vi "Track Overflow.vi"(2 "reset":bool, 5 "overflow in":bool[](array[boolean])=[FALSE, FALSE, FALSE, FALSE, FALSE, FALSE, FALSE, FALSE, FALSE, FALSE, FALSE, FALSE, FALSE, FALSE, FALSE, FALSE], 7 "input valid":bool, 9 "latch overflow status":bool) -> (10 "overflow detected":bool)   [LabVIEW 2018, in "GettingStarted_5774_FPGA.lvlib"]
doc: "Tracks the overflow status.\n\nA rising edge on the <B>latch overflow status</B> input updates the <B>overflow detected</B> output: this output is set to true if an overflow was detected since the last update."
uses:
  GettingStarted_5774_FPGA.lvlib
  <instrlib>/_niInstr/Basic Elements/v1/FPGA/niInstr Basic Elements v1 FPGA.lvlib
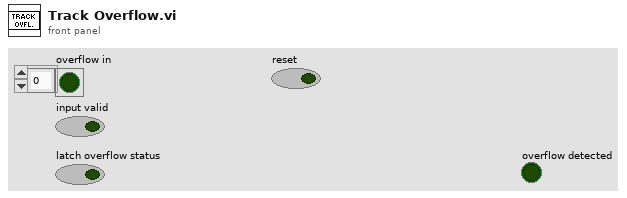
[diagram p1: front panel]
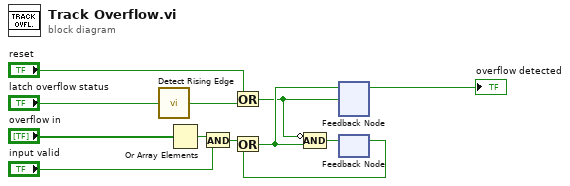
[diagram p0: block diagram]
diagram:
  n1 = call <instrlib>:"Detect Rising Edge.vi"("signal"="latch overflow status") -> ("edge detected"=w1:bool)  [unwired: 14 in]
  n2 = Or Array Elements(Boolean array="overflow in") -> (logical OR=w11:bool)
  n3 = And(x=w11, y="input valid") -> (x .and. y?=w9:bool)
  n4 = Or(x="reset", y=w1) -> (x .or. y?=w4:bool)
  n5 = feedback #1() -> (→"overflow detected":bool)  [unwired: 1 in]
  n6 = feedback #2() -> (w8:bool)  [unwired: 1 in]
  n7 = Or(x=w9, y=w8) -> (x .or. y?=w5:bool)
  n8 = Compound Arithmetic op=AND(invert w4, w5) -> (w3:bool)
  n9 = feedback-in #1(w5, w4) -> ()
  n10 = feedback-in #2(w3) -> ()
